vi "Begin (Christian Colglazier's conflicted copy 2013-08-17).vi"(11 "Image Size":T1=enum."160x120") -> (0 "error out":errorcluster)   [LabVIEW 2012]
doc: "Called before other user functions, this VI is expected to open initial I/O refnums, load in file data, and do all program initialization. Notice that the <B>error out</B> terminal is simply used for data flow. Wiring it to other structures or subVIs ensures that this VI runs first."
uses:
  <vilib>/Rock Robotics/WPI/Camera/WPI_CameraImageSize.ctl
  <vilib>/Rock Robotics/SystemInterfaces/DIO/FPGA_DIOPWMChannel.ctl
  <vilib>/Rock Robotics/WPI/Camera/WPI_CameraWhite Balance Values.ctl
  <vilib>/Rock Robotics/WPI/Camera/WPI_CameraExposure Values.ctl
  <vilib>/Rock Robotics/WPI/Camera/WPI_CameraFrameRate.ctl
  <vilib>/Rock Robotics/WPI/SafetyOutput/WPI_SafetyOutputConfigMenu.ctl
  <vilib>/Rock Robotics/WPI/DriverStation/WPI_DriverStationRobotMode2.ctl
  <vilib>/Rock Robotics/WPI/Joystick/WPI_JoystickDeviceEnum.ctl
  <vilib>/Rock Robotics/SystemInterfaces/DIO/FPGA_DIOChannel.ctl
  <vilib>/Rock Robotics/SystemInterfaces/DIO/FPGA_DIORelayChannel.ctl
  <vilib>/Rock Robotics/WPI/Solenoid/WPI_SolenoidChannel.ctl
  <vilib>/Rock Robotics/SystemInterfaces/AI/FPGA_AIChannel.ctl
  Robot Global Data.vi
  <vilib>/Rock Robotics/WPI/RobotDrive/WPI_RobotDriveOpen4MotorWithJaguar.vi
  <vilib>/Rock Robotics/WPI/MotorControl/WPI_MotorControlOpen Talon.vi
  <vilib>/Rock Robotics/WPI/Solenoid/WPI_SolenoidOpenDouble.vi
  <vilib>/Rock Robotics/WPI/Compressor/WPI_CompressorGetSetRefNum.vi
  <vilib>/Rock Robotics/WPI/RobotDrive/WPI_RobotDriveOpen2MotorWithJaguar.vi
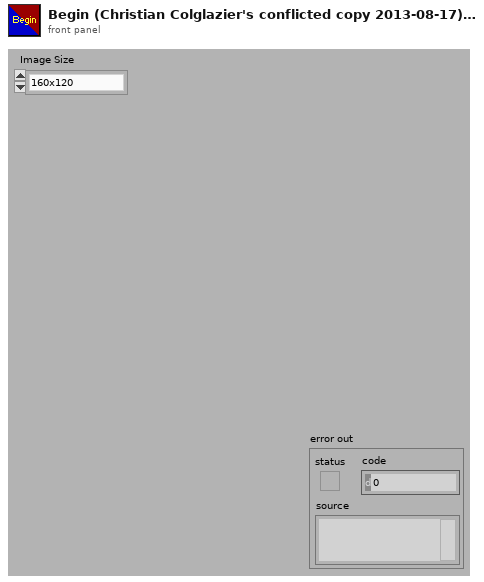
[diagram p1: front panel]
types:
  T1 = typedef "WPI_CameraImageSize.ctl" = enum16{"640x480", "320x240", "160x120"}
  T2 = typedef "FPGA_AIChannel.ctl" = enum8{"AI 1", "AI 2", "AI 3", "AI 4", "AI 5", "AI 6", "AI 7", "AI 8", "Invalid"}
  T3 = typedef "FPGA_DIOPWMChannel.ctl" = enum8{"PWM 1", "PWM 2", "PWM 3", "PWM 4", "PWM 5", "PWM 6", "PWM 7", "PWM 8", "PWM 9", "PWM 10", "Invalid"}
  T4 = typedef "FPGA_DIOChannel.ctl" = enum8{"DIO 1", "DIO 2", "DIO 3", "DIO 4", "DIO 5", "DIO 6", "DIO 7", "DIO 8", "DIO 9", "DIO 10", "DIO 11", "DIO 12", "DIO 13", "DIO 14", "Invalid"}
  T5 = typedef "WPI_SolenoidChannel.ctl" = enum8{"Solenoid 1", "Solenoid 2", "Solenoid 3", "Solenoid 4", "Solenoid 5", "Solenoid 6", "Solenoid 7", "Solenoid 8", "Invalid"}
  T6 = typedef "FPGA_DIORelayChannel.ctl" = enum8{"Relay 1", "Relay 2", "Relay 3", "Relay 4", "Relay 5", "Relay 6", "Relay 7", "Relay 8", "Invalid"}
  T7 = typedef "WPI_JoystickDeviceEnum.ctl" = enum16{"USB 1", "USB 2", "USB 3", "USB 4", "Kinect 1", "Kinect 2"}
  T8 = typedef "WPI_DriverStationRobotMode2.ctl" = enum16{"Autonomous Disabled", "Autonomous Enabled", "Teleop Disabled", "Teleop Enabled", "Timeout", "Finish", "Test Disabled", "Test Enabled"}
  T9 = typedef "WPI_SafetyOutputConfigMenu.ctl" = enum16{"Enable", "Disable"}
  T10 = typedef "WPI_CameraFrameRate.ctl" = u32
  T11 = typedef "WPI_CameraExposure Values.ctl" = enum16{"Auto", "Flicker-free 50 Hz", "Flicker-free 60 Hz", "Hold current"}
  T12 = typedef "WPI_CameraWhite Balance Values.ctl" = enum16{"Auto", "Fixed indoor", "Fixed outdoor 1", "Fixed outdoor 2", "Fixed fluorescent 1", "Fixed fluorescent 2", "Hold current"}
  T13 = typedef "WPI_RobotDriveDevRef.ctl" = cluster{"DevStatus":errorcluster, "Motors[]":T14[], "Square Inputs":bool, "Max Output":dbl, "Isochronous":bool}
  T14 = typedef "WPI_MotorControlDeviceRef.ctl" = cluster{"DeviceStatus":errorcluster, "Type":enum16{"PWM", "CAN"}, "PWM":cluster{"Digital Module":T15, "PWM Channel":T3, "DeadBand":T16}, "CAN":cluster{"Device Number":u8, "Control Mode":T17, "Semaphore":T18, "Max Vout":dbl}, "Invert":bool, "TransformRef":T19, "InvTransformRef":T19}
  T15 = typedef "FPGA_TypedefDigitalModule.ctl" = enum16{"Digital Module 1", "Digital Module 2"}
  T16 = typedef "WPI_PWMDeadband.ctl" = cluster{"Name":string, "maxPositivePwm":i32, "minPositivePwm":i32, "centerPwm":i32, "maxNegativePwm":i32, "minNegativePwm":i32, "angularRange":u16}
  T17 = typedef "WPI_CANJaguar_ControlMode.ctl" = enum8{"Percent VBus", "Current", "Speed", "Position", "Voltage"}
  T18 = typedef "Semaphore RefNum" = refnum<k1>
  T19 = typedef "WPI_PWMTransform_ConPane.ctl" = refnum<vi>
  T20 = typedef "WPI_ServoDeviceRef.ctl" = cluster{"DeviceStatus":errorcluster, "Digital Module":T15, "PWM Channel":T3, "DeadBand":T16}
  T21 = typedef "WPI_CameraDevRef.ctl" = cluster{"Camera Address":string, "CameraStatus":errorcluster, "Acquire Image Notifier":refnum<notifier>}
  T22 = typedef "WPI_JoystickDevRef.ctl" = cluster{"Device":T7}
  T23 = typedef "WPI_SolenoidDevRef.ctl" = cluster{"DevStatus":errorcluster, "Solenoid Module":T24, "Forward Solenoid Channel":T5, "Reverse Solenoid Channel":T5}
  T24 = typedef "FPGA_TypedefSolenoidModule.ctl" = enum16{"Solenoid Module 1", "Solenoid Module 2"}
  T25 = typedef "WPI_AnalogChannelDevRef.ctl" = cluster{"DevStatus":errorcluster, "Analog Module":T26, "Analog Channel":T2}
  T26 = typedef "FPGA_TypedefAnalogModule.ctl" = enum16{"Analog Module 1", "Analog Module 2"}
  T27 = typedef "WPI_CompressorDevRef.ctl" = cluster{"DevStatus":errorcluster, "DigitalInputDevRef":T28, "RelayDevRef":T29}
  T28 = typedef "WPI_DigitalInputDevRef.ctl" = cluster{"DevStatus":errorcluster, "DIO Channel":T4, "Digital Module":T15}
  T29 = typedef "WPI_RelayDevRef.ctl" = cluster{"DevStatus":errorcluster, "Relay Channel":T6, "Digital Module":T15, "Relay Direction":T30}
  T30 = typedef "WPI_RelayDirection.ctl" = enum16{"Both directions", "Forward only", "Reverse only"}
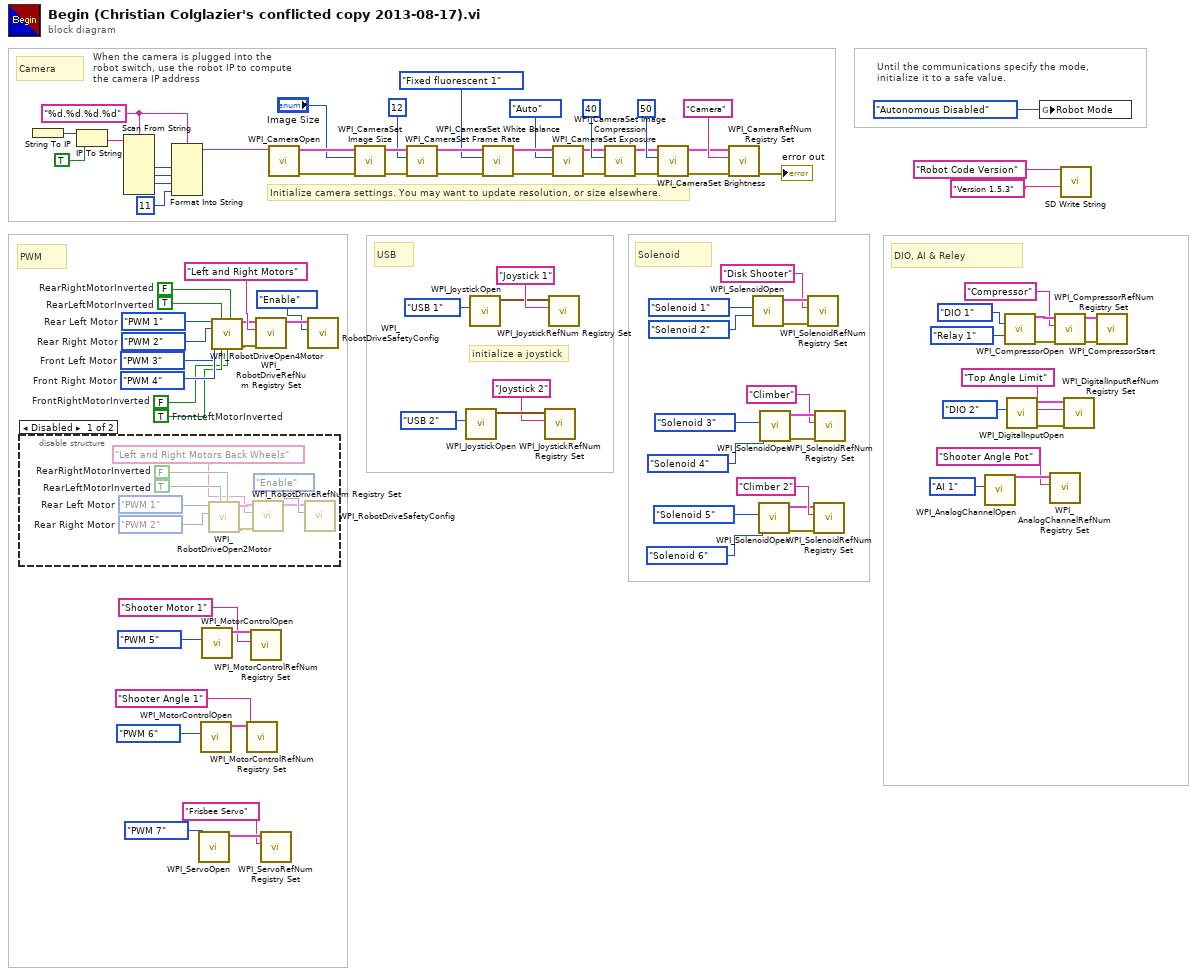
[diagram p0: block diagram]
diagram:
  w45 = TRUE  # FrontLeftMotorInverted
  w44 = FALSE  # FrontRightMotorInverted
  w47 = FPGA_DIOPWMChannel."PWM 4"  # Front Right Motor
  w46 = FPGA_DIOPWMChannel."PWM 3"  # Front Left Motor
  w62 = "%d.%d.%d.%d" ("format string")
  w48 = FPGA_DIOPWMChannel."PWM 2"  # Rear Right Motor
  w49 = FPGA_DIOPWMChannel."PWM 1"  # Rear Left Motor
  w51 = TRUE  # RearLeftMotorInverted
  w50 = FALSE  # RearRightMotorInverted
  # "Camera"
  # "DIO, AI & Reley"
  # "PWM"
  # "Solenoid"
  # "USB"
  # "initialize a joystick"
  # "Until the communications specify the mode,\ninitialize it to a safe value."
  # "When the camera is plugged into the\nrobot switch, use the robot IP to compute\nthe camera IP address"
  # "Initialize camera settings. You may want to update resolution, or size elsewhere."
  n1 = disable-structure shown="Disabled" {
    frame Disabled {
      w100 = FPGA_DIOPWMChannel."PWM 2"  # Rear Right Motor
      w99 = FPGA_DIOPWMChannel."PWM 1"  # Rear Left Motor
      w97 = TRUE  # RearLeftMotorInverted
      w98 = FALSE  # RearRightMotorInverted
      n2 = call-poly <vilib>:"WPI_RobotDriveOpen2Motor.vi"("Right Motor Inverted"=w98, "Left Motor Inverted"=w97, "Right Motor"=w100, "Left Motor"=w99) -> ("error out"=w95:errorcluster, "RobotDriveDevRef"=w96:T13)  [unwired: 6 in]
      n3 = call <vilib>:"WPI_RobotDriveRefNum Registry Set.vi"("error in (no error)"=w95, "refnum name"="Left and Right Motors Back Wheels", "RobotDriveDevRef"=w96) -> ("RobotDriveDevRef"=w93:T13)  [unwired: 8 out]
      n4 = call <vilib>:"WPI_RobotDriveSafetyConfig.vi"("mode"=WPI_SafetyOutputConfigMenu."Enable", "RobotDriveDevRef"=w93) -> ()  [unwired: 8 in, 2 out]
    }
    frame Enabled {
    }
  }
  n5 = String To IP() -> (0:w69:u32)  [unwired: 1 in]
  n6 = IP To String(1:TRUE ("dot notation? (F)"), 2:w69) -> (0:w67:string)
  n7 = Scan From String(format string=w62, input string=w67) -> (output 1=w66:i32, output 2=w65:i32, output 3=w64:i32)  [unwired: 7 in, 3 out]
  n8 = Format Into String(format string=w62, w66, w65, w64, 11 ("Compression")) -> (resulting string=w58:string)  [unwired: 2 in, 1 out]
  n9 = call <vilib>:"WPI_ServoOpen.vi"("PWM Channel"=FPGA_DIOPWMChannel."PWM 7") -> ("ServoDeviceRef"=w6:T20)  [unwired: 9 in, 1 out]
  n10 = call-poly <vilib>:"WPI_MotorControlOpen.vi"("PWM Channel"=FPGA_DIOPWMChannel."PWM 6") -> ("MotorControlDeviceRef"=w39:T14)  [unwired: 9 in, 1 out]
  n11 = call-poly <vilib>:"WPI_MotorControlOpen.vi"("PWM Channel"=FPGA_DIOPWMChannel."PWM 5") -> ("MotorControlDeviceRef"=w42:T14)  [unwired: 9 in, 1 out]
  n12 = call-poly <vilib>:"WPI_RobotDriveOpen4Motor.vi"("Rear Left Motor"=w49, "Rear Left Motor Inverted"=w51, "Rear Right Motor Inverted"=w50, "Rear Right Motor"=w48, "Front Left Motor"=w46, "Front Right Motor"=w47, "Front Left Motor Inverted"=w45, "Front Right Motor Inverted"=w44) -> ("RobotDriveDevRef"=w52:T13, "error out"=w53:errorcluster)  [unwired: 6 in]
  n13 = call <vilib>:"WPI_MotorControlRefNum Registry Set.vi"("refnum name"="Shooter Angle 1", "MotorControlDevRef"=w39) -> ()  [unwired: 8 in, 2 out]
  n14 = call <vilib>:"WPI_MotorControlRefNum Registry Set.vi"("refnum name"="Shooter Motor 1", "MotorControlDevRef"=w42) -> ()  [unwired: 8 in, 2 out]
  n15 = call <vilib>:"WPI_RobotDriveRefNum Registry Set.vi"("error in (no error)"=w53, "refnum name"="Left and Right Motors", "RobotDriveDevRef"=w52) -> ("RobotDriveDevRef"=w61:T13)  [unwired: 8 out]
  n16 = call <vilib>:"WPI_ServoRefNum Registry Set.vi"("refnum name"="Frisbee Servo", "ServoDeviceRef"=w6) -> ()  [unwired: 8 in, 2 out]
  n17 = call <vilib>:"WPI_CameraOpen.vi"("Camera Address"=w58) -> ("error out"=w81:errorcluster, "CameraDevRef"=w82:T21)  [unwired: 1 in, 8 out]
  n18 = call <vilib>:"WPI_RobotDriveSafetyConfig.vi"("mode"=WPI_SafetyOutputConfigMenu."Enable", "RobotDriveDevRef"=w61) -> ()  [unwired: 8 in, 2 out]
  n19 = call <vilib>:"WPI_CameraSet Image Size.vi"("error in (no error)"=w81, "Image Size"="Image Size", "CameraDevRef"=w82) -> ("error out"=w80:errorcluster, "CameraDevRef Out"=w83:T21)  [unwired: 7 out]
  n20 = call <vilib>:"WPI_CameraSet Frame Rate.vi"("error in (no error)"=w80, "Frame Rate (fps)"=T10 12, "CameraDevRef"=w83) -> ("error out"=w79:errorcluster, "CameraDevRef Out"=w85:T21)  [unwired: 7 out]
  n21 = call <vilib>:"WPI_JoystickOpen.vi"("JoystickDevice"=WPI_JoystickDeviceEnum."USB 2") -> ("JoystickDevRef"=w36:T22)  [unwired: 10 in]
  n22 = call <vilib>:"WPI_JoystickOpen.vi"("JoystickDevice"=WPI_JoystickDeviceEnum."USB 1") -> ("JoystickDevRef"=w56:T22)  [unwired: 10 in]
  n23 = call <vilib>:"WPI_CameraSet White Balance.vi"("error in (no error)"=w79, "White Balance"=WPI_CameraWhite_Balance_Values."Fixed fluorescent 1", "CameraDevRef"=w85) -> ("error out"=w78:errorcluster, "CameraDevRef Out"=w84:T21)  [unwired: 7 out]
  n24 = call <vilib>:"WPI_JoystickRefNum Registry Set.vi"("refnum name"="Joystick 2", "JoystickDevRef"=w36) -> ()  [unwired: 8 in, 2 out]
  n25 = call <vilib>:"WPI_JoystickRefNum Registry Set.vi"("refnum name"="Joystick 1", "JoystickDevRef"=w56) -> ()  [unwired: 8 in, 2 out]
  n26 = call <vilib>:"WPI_CameraSet Exposure.vi"("error in (no error)"=w78, "Exposure"=WPI_CameraExposure_Values."Auto", "CameraDevRef"=w84) -> ("error out"=w77:errorcluster, "CameraDevRef Out"=w87:T21)  [unwired: 7 out]
  n27 = call <vilib>:"WPI_CameraSet Image Compression.vi"("error in (no error)"=w77, "Compression"=40, "CameraDevRef"=w87) -> ("error out"=w76:errorcluster, "CameraDevRef Out"=w86:T21)  [unwired: 7 out]
  n28 = call <vilib>:"WPI_CameraSet Brightness.vi"("error in (no error)"=w76, "Brightness"=50, "CameraDevRef"=w86) -> ("error out"=w74:errorcluster, "CameraDevRef Out"=w75:T21)  [unwired: 7 out]
  n29 = call <vilib>:"WPI_CameraRefNum Registry Set.vi"("error in (no error)"=w74, "refnum name"="Camera", "CameraDevRef"=w75) -> ("error out"=→"error out":errorcluster)  [unwired: 8 out]
  n30 = call-poly <vilib>:"WPI_SolenoidOpen.vi"("Reverse Solenoid Channel"=WPI_SolenoidChannel."Solenoid 2" ("Forward Solenoid Channel"), "Forward Solenoid Channel"=WPI_SolenoidChannel."Solenoid 1" ("Solenoid Channel")) -> ("error out"=w26:errorcluster, "SolenoidDevRef"=w25:T23)  [unwired: 8 in]
  n31 = call-poly <vilib>:"WPI_SolenoidOpen.vi"("Reverse Solenoid Channel"=WPI_SolenoidChannel."Solenoid 6" ("Forward Solenoid Channel"), "Forward Solenoid Channel"=WPI_SolenoidChannel."Solenoid 5" ("Solenoid Channel")) -> ("error out"=w14:errorcluster, "SolenoidDevRef"=w13:T23)  [unwired: 8 in]
  n32 = call-poly <vilib>:"WPI_SolenoidOpen.vi"("Reverse Solenoid Channel"=WPI_SolenoidChannel."Solenoid 4" ("Forward Solenoid Channel"), "Forward Solenoid Channel"=WPI_SolenoidChannel."Solenoid 3" ("Solenoid Channel")) -> ("error out"=w21:errorcluster, "SolenoidDevRef"=w22:T23)  [unwired: 8 in]
  n33 = call <vilib>:"WPI_SolenoidRefNum Registry Set.vi"("error in (no error)"=w26, "refnum name"="Disk Shooter", "SolenoidDevRef"=w25) -> ()  [unwired: 7 in, 2 out]
  n34 = call <vilib>:"WPI_SolenoidRefNum Registry Set.vi"("error in (no error)"=w14, "refnum name"="Climber 2", "SolenoidDevRef"=w13) -> ()  [unwired: 7 in, 2 out]
  n35 = call <vilib>:"WPI_SolenoidRefNum Registry Set.vi"("error in (no error)"=w21, "refnum name"="Climber", "SolenoidDevRef"=w22) -> ()  [unwired: 7 in, 2 out]
  n36 = call <vilib>:"WPI_AnalogChannelOpen.vi"("Analog Channel"=FPGA_AIChannel."AI 1") -> ("AIDeviceRef"=w3:T25)  [unwired: 9 in, 1 out]
  n37 = call <vilib>:"WPI_CompressorOpen.vi"("Pressure Switch DIO Channel"=FPGA_DIOChannel."DIO 1", "Relay Channel"=FPGA_DIORelayChannel."Relay 1") -> ("CompressorDevRef"=w32:T27, "error out"=w29:errorcluster)  [unwired: 12 in]
  n38 = call <vilib>:"WPI_DigitalInputOpen.vi"("DIO Channel"=FPGA_DIOChannel."DIO 2") -> ("error out"=w12:errorcluster, "DigitalInputDevRef"=w11:T28)  [unwired: 9 in]
  n39 = global write "Robot Global Data.vi" "Robot Mode"(WPI_DriverStationRobotMode2."Autonomous Disabled" ("Robot Mode")) -> ()
  n40 = call <vilib>:"WPI_AnalogChannelRefNum Registry Set.vi"("refnum name"="Shooter Angle Pot", "AIDeviceRef"=w3) -> ()  [unwired: 8 in, 2 out]
  n41 = call <vilib>:"WPI_CompressorRefNum Registry Set.vi"("error in (no error)"=w29, "refnum name"="Compressor", "CompressorDevRef"=w32) -> ("error out"=w34:errorcluster, "CompressorDevRef"=w33:T27)  [unwired: 7 in]
  n42 = call <vilib>:"SD Write String.vi"("String"="Version 1.5.3", "Name"="Robot Code Version") -> ()  [unwired: 8 in, 2 out]
  n43 = call <vilib>:"WPI_DigitalInputRefNum Registry Set.vi"("error in (no error)"=w12, "refnum name"="Top Angle Limit", "DigitalInputDevRef"=w11) -> ()  [unwired: 7 in, 2 out]
  n44 = call <vilib>:"WPI_CompressorStart.vi"("error in (no error)"=w34, "CompressorDevRef"=w33) -> ()  [unwired: 8 in, 2 out]
